vi "叶绿素a单位换算.vi"(11 "叶绿素a显示":T1) -> (1 "数据标识":string, 2 "检测值1.单位":string, 3 "测量值":sgl)   [LabVIEW 2022 SP3, in "斯坦道多参数.lvlib"]
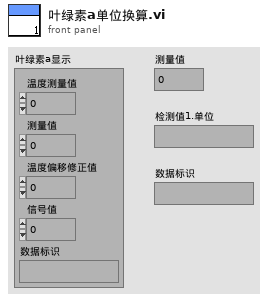
[diagram p1: front panel]
types:
  T1 = cluster{"温度测量值":sgl, "测量值":sgl, "温度偏移修正值":sgl, "信号值":sgl, "数据标识":string}
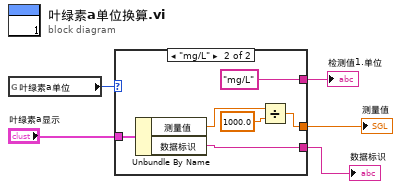
[diagram p0: block diagram]
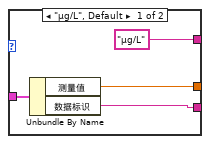
[diagram p2: hidden frame]
diagram:
  n1 = global read "断电保存变量.vi" "叶绿素a单位"() -> (w2:enum16{"μg/L", "mg/L"})
  n2 = case shown="\"mg/L\"" w2 {
    tunnel: "叶绿素a显示" -> [w9 w15]
    tunnel: ["μg/L" ("检测值1.单位") "mg/L" ("检测值1.单位")] -> w3
    tunnel: [w7 w11] -> w4
    tunnel: [w6 w12] -> w5
    frame "μg/L", Default {
      n3 = Unbundle By Name(w9) -> ("测量值"=w7:sgl, "数据标识"=w6:string)
    }
    frame "mg/L" {
      n4 = Unbundle By Name(w15) -> ("测量值"=w13:sgl, "数据标识"=w12:string)
      n5 = Divide(x=w13, y=sgl 1000.0) -> (x/y=w11:sgl)
    }
  }
  "数据标识" <- w5
  "测量值" <- w4
  "检测值1.单位" <- w3
